vi "Store Manual Observer.vi"(8 "error in (no error)":errorcluster, 10 "Observer In":refnum<class "Observer.lvclass">, 11 "Vessel in":refnum<class "Vessel.lvclass">) -> (0 "error out":errorcluster, 3 "Vessel out":refnum<class "Vessel.lvclass">)   [LabVIEW 2014, in "Vessel.lvclass"]
uses:
  Vessel.lvclass
  Observer/Observer.lvclass
  Supervisor/Supervisor.lvclass
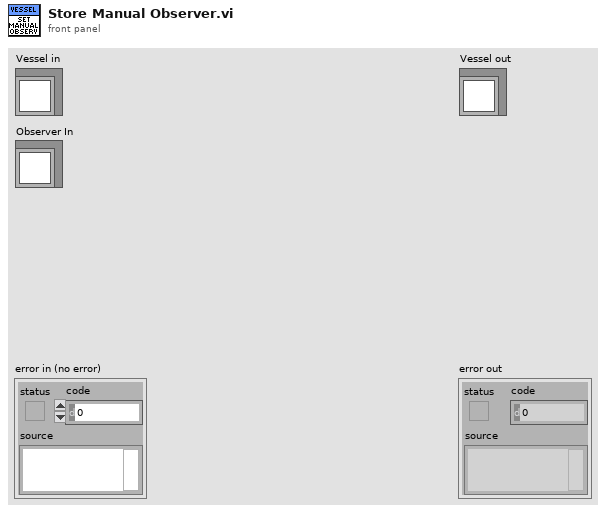
[diagram p1: front panel]
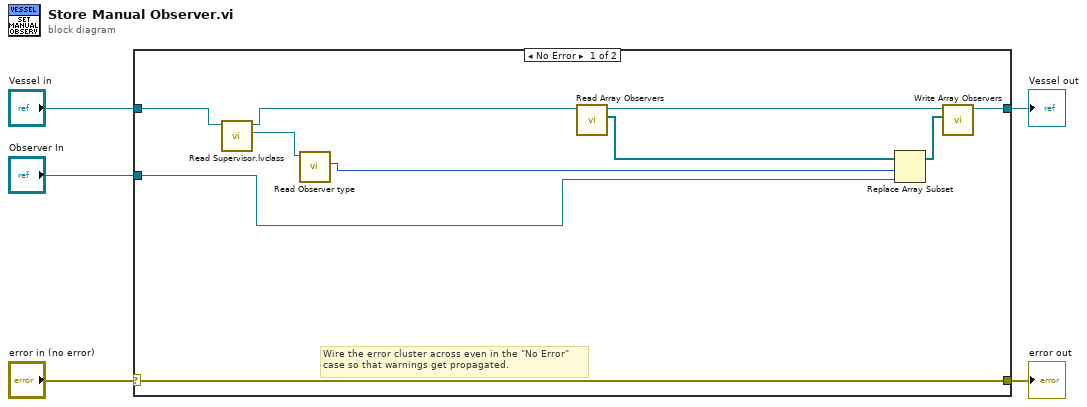
[diagram p0: block diagram]
diagram:
  n1 = case shown="No Error" "error in (no error)" {
    selector: "error in (no error)" -> [w15 w17]
    tunnel: [w15 w17] -> w4
    tunnel: [w11 w16] -> w2
    tunnel: "Vessel in" -> [w14 w16]
    tunnel: "Observer In" -> [w8 _]
    frame No Error {
      # "Wire the error cluster across even in the \"No Error\"\ncase so that warnings get propagated."
      n2 = call "Read Supervisor.lvclass.vi"("Vessel in"=w14) -> ("Supervisor.lvclass"=w7:refnum<class "Supervisor.lvclass">, "Vessel out"=w12:refnum<class "Vessel.lvclass">)  [unwired: 8 in, 1 out]
      n3 = call-dynamic "Read Observer type.vi"("Supervisor in"=w7) -> ("Observer type"=w6:i16)  [unwired: 8 in, 2 out]
      n4 = call-dynamic "Read Array Observers.vi"("Vessel in"=w12) -> ("Array Observers"=w13:refnum<class "Observer.lvclass">[], "Vessel out"=w9:refnum<class "Vessel.lvclass">)  [unwired: 8 in, 1 out]
      n5 = Replace Array Subset(array=w13, new element=w8, index=w6) -> (w10:refnum<class "Observer.lvclass">[])
      n6 = call-dynamic "Write Array Observers.vi"("Array Observers"=w10, "Vessel in"=w9) -> ("Vessel out"=w11:refnum<class "Vessel.lvclass">)  [unwired: 8 in, 1 out]
    }
    frame Error {
    }
  }
  "error out" <- w4
  "Vessel out" <- w2
